vi "PE_IoTSerialProcessor.vi"() -> ()   [LabVIEW 2016]
uses:
  SerialSupport/Serial - Settings.ctl
  SerialSupport/Serial - XON-XOFF Characters.ctl
  SerialSupport/Serial - ASCII Characters.ctl
  <vilib>/Instr/_visa.llb/VISA Configure Serial Port (Instr).vi
  database/database.lvlib
panel:
  in  "持久化开关":bool=TRUE
  in  "参考电阻_AgNW":dbl
  in  "总压降":dbl=65535.0
  in  "参考电阻_ITO":dbl
  in  "JSON parser":T1
  in  "TestId":string
  out "波形图表 2":dynamicdata(graph)
  out "json error":errorcluster caption="JSON Error"
  in  "dataLabel":string
  in  "msg_id":dbl
  out "CtrlCmdMsg":string
  out "串口信息发送持久化":bool=TRUE
  out "串口信息发送":bool=TRUE
  out "UDP发送持久化":bool=TRUE
  out "TCP发送持久化":bool=TRUE
  out "串口接收持久化":bool=TRUE
  in  "串口发送按钮":bool
  in  "终止符":u8=10 format="%.0x"
  in  "终止符时结束写入？":bool=TRUE
  in  "VISA资源名称":refnum<visa-resource-name>="COM3"
  in  "XON/XOFF字符":T2={"XON"=enum."DC1", "XOFF"=enum."DC3"}
  in  "串口设置":T4={"波特率"=115200, "数据位"=8, "校验"=enum."None", "停止位"=10, "流控制"=0} {"流控制" items=["无"=0, "XON/XOFF"=1, "RTS/CTS"=2, "DTR/DSR"=4]; "停止位" items=["1.0"=10, "1.5"=15, "2.0"=20]; "数据位" min=5 max=8 step=1; "波特率" items=["75"=75, "110"=110, "134"=134, "150"=150, "300"=300, "600"=600, "1200"=1200, "1800"=1800, "2400"=2400, "4800"=4800, "7200"=7200, "9600"=9600, "14400"=14400, "19200"=19200, "28800"=28800, "38400"=38400, "56000"=56000, "57600"=57600, "115200"=115200, "128000"=128000, "230400"=230400]}
  in  "终止符时结束读取？":bool=TRUE
  in  "读取":bool=TRUE
  in  "串口停止":bool
  in  "串口发送命令":string="{\"cmd\":\"CT_ON\",\"id\":\"C_FR\",on:true}"
  out "串口信息":string
  in  "串口最大字节":u32=1000
  out "当前指令":string
  # "Smart thermalchromic window monitoring"
  # "Test Information Setting"
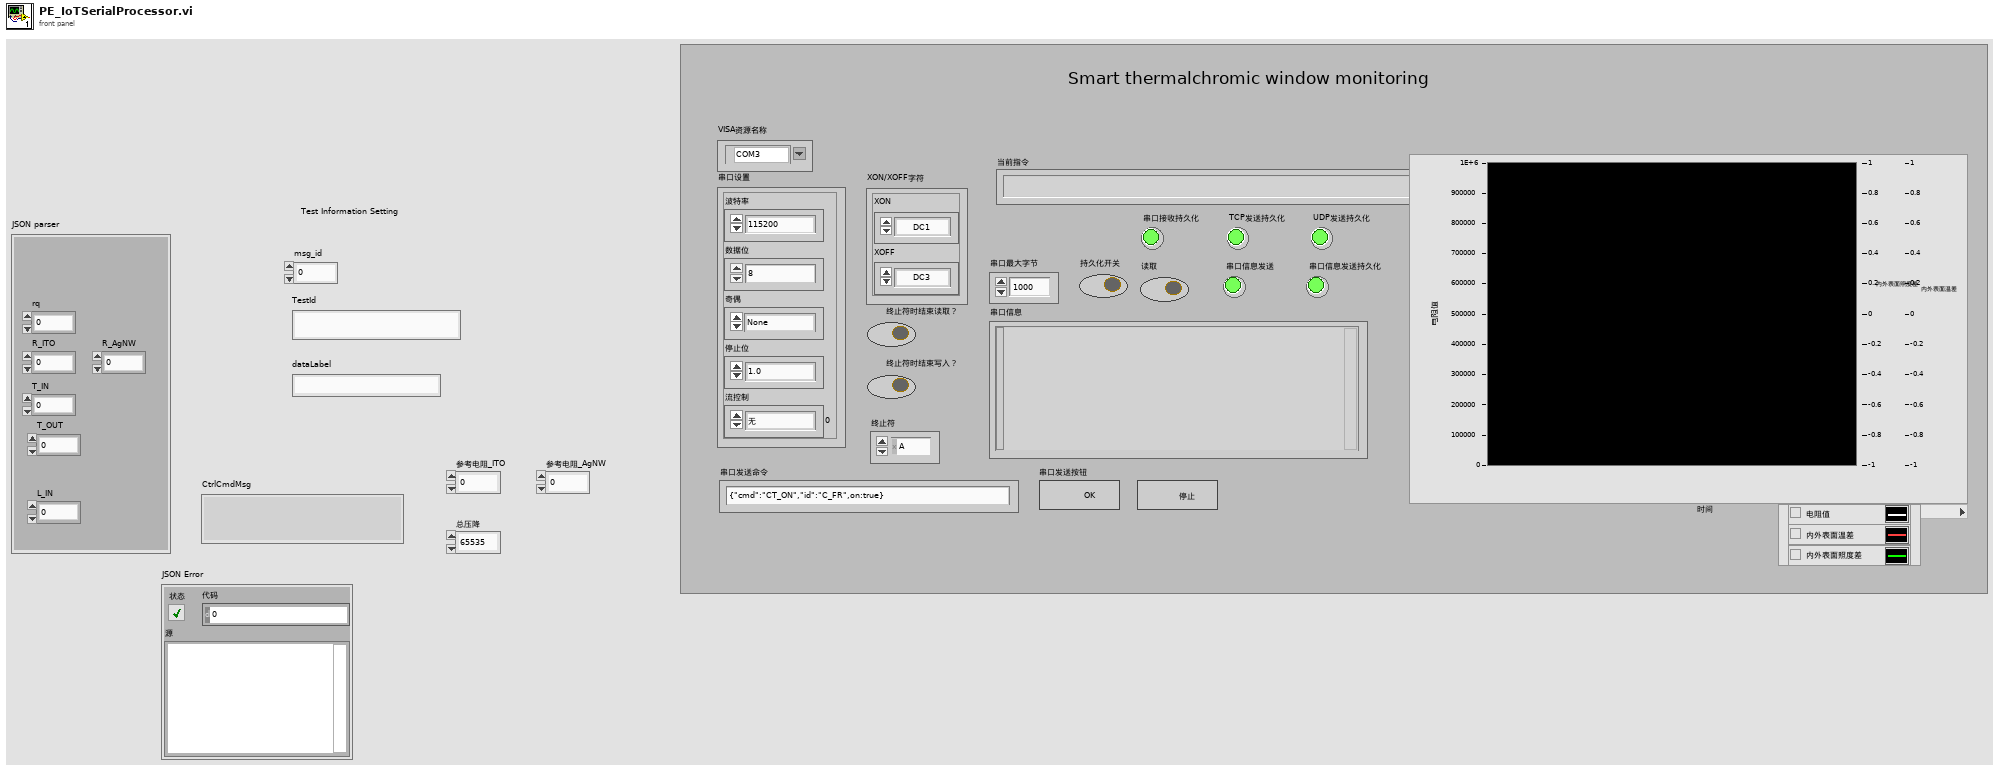
[diagram p1: front panel]
types:
  T1 = cluster{"rq":dbl, "R_ITO":dbl, "T_IN":dbl, "T_OUT":dbl, "R_AgNW":dbl, "L_IN":dbl}
  T2 = typedef "Serial - XON-XOFF Characters.ctl" = cluster{"XON":T3, "XOFF":T3}
  T3 = typedef "Serial - ASCII Characters.ctl" = enum16{"NUL", "SOH", "STX", "ETX", "EOT", "ENQ", "ACK", "BEL", "BS", "HT", "LF", "VT", "FF", "CR", "SO", "SI", "DLE", "DC1", "DC2", "DC3", "DC4", "NAK", "SYN", "ETB", "CAN", "EM", "SUB", "ESC", "FS", "GS", "RS", "US", "SP", "!", "\"", "#", "$", "%", "&", "'", "(", ")", "*", "+", ",", "- (-)", ".", "/", "0", "1", "2", "3", "4", "5", "6", "7", "8", "9", ":", ";", "<", "=", ">", "?", "@", "A", "B", "C", "D", "E", "F", "G", "H", "I", "J", "K", "L", "M", "N", "O", "P", "Q", "R", "S", "T", "U", "V", "W", "X", "Y", "Z", "[", "\\", "]", "^", "_", "`", "a", "b", "c", "d", "e", "f", "g", "h", "i", "j", "k", "l", "m", "n", "o", "p", "q", "r", "s", "t", "u", "v", "w", "x", "y", "z", "{", "|", "}", "~"}
  T4 = typedef "Serial - Settings.ctl" = cluster{"波特率":u32, "数据位":u16, "校验":enum16{"None", "Odd", "Even", "Mark", "Space"}, "停止位":u16, "流控制":u16}
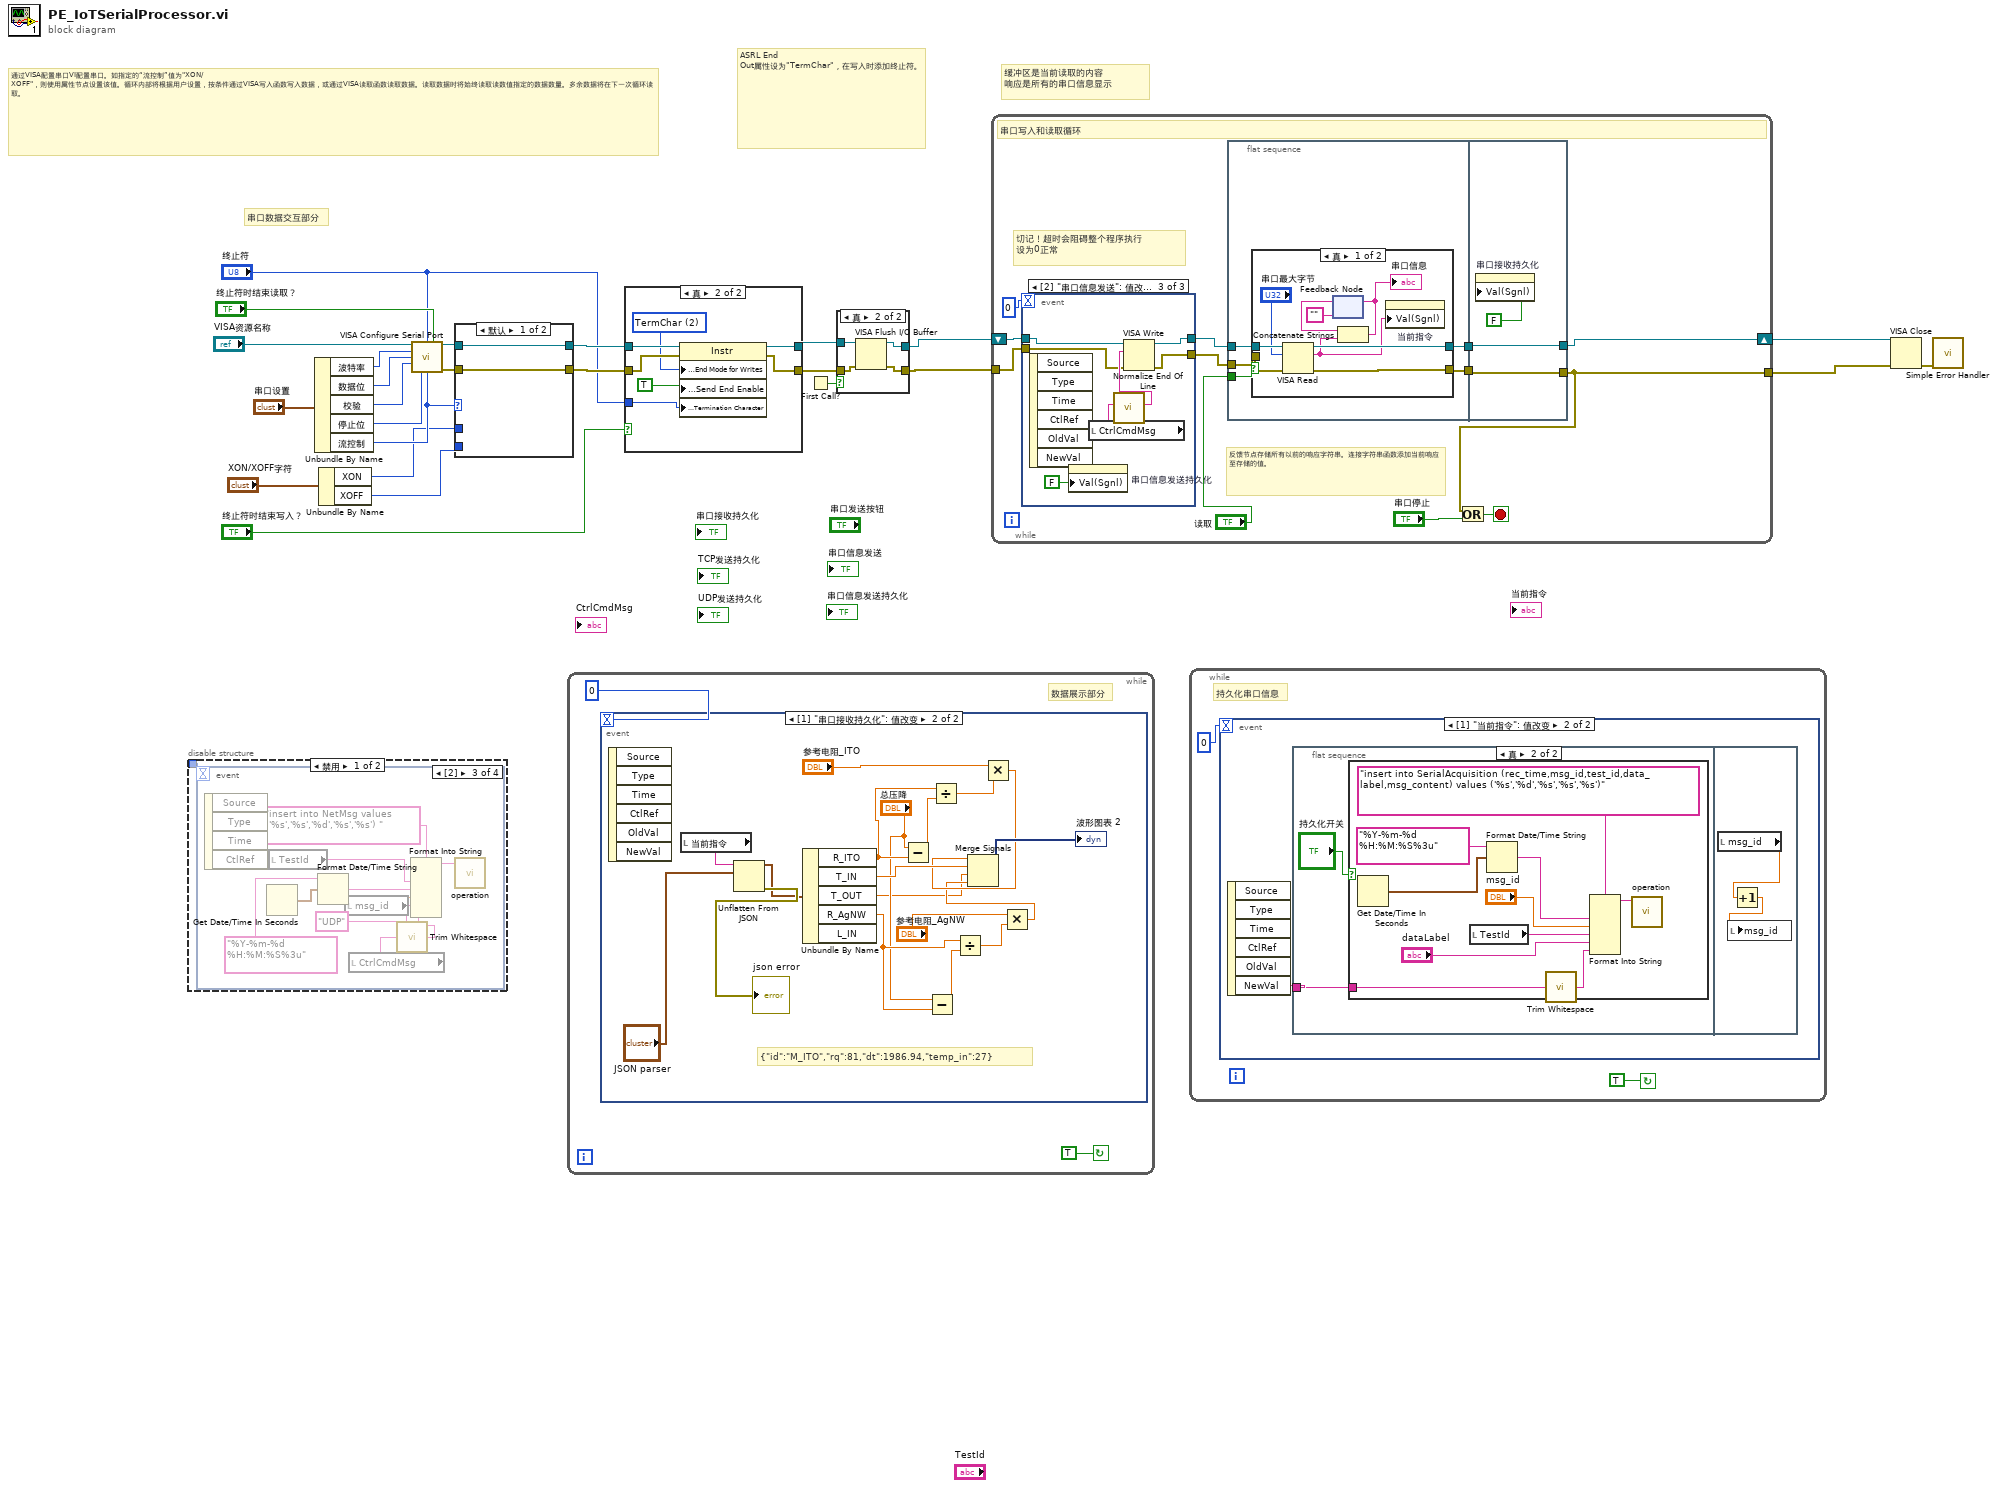
[diagram p0: block diagram]
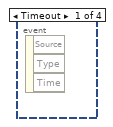
[diagram p2: hidden frame]
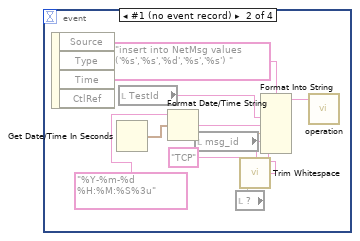
[diagram p3: hidden frame]
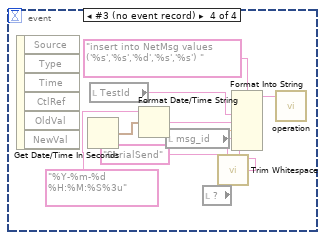
[diagram p4: hidden frame]
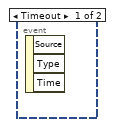
[diagram p6: hidden frame]
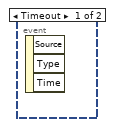
[diagram p8: hidden frame]
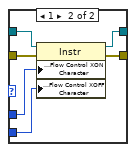
[diagram p11: hidden frame]
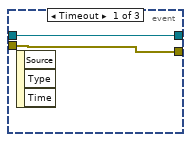
[diagram p13: hidden frame]
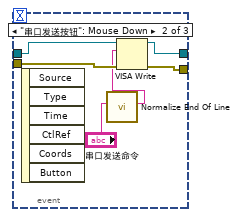
[diagram p14: hidden frame]
diagram:
  # "串口数据交互部分"
  # "缓冲区是当前读取的内容\n响应是所有的串口信息显示"
  # "ASRL End Out属性设为\"TermChar\"，在写入时添加终止符。"
  # "通过VISA配置串口VI配置串口。如指定的“流控制”值为\"XON/XOFF\"，则使用属性节点设置该值。循环内部将根据用户设置，按条件通过VISA写入函数写入数据，或通过VISA读取函数读取数据。读取数据时将始终读取读数值指定的数据数量。多余数据将在下一次循环读取。"
  n1 = disable-structure shown="禁用" {
    disable-tunnel: _ -> [w26 _]
    frame Disabled {
      n2 = event shown="[2]" {
        selector: _ -> [_ _ _ _]
        dyn-events: _ -> [_ _ _ _]
        timeout: w26 -> [_ _ _ _]
        event Timeout {
          n3 = event-data() -> ()  [unwired: 1 in, 3 out]
        }
        event #1 (no event record) {
          n4 = event-data() -> ()  [unwired: 1 in, 4 out]
          n5 = Get Date/Time In Seconds() -> (seconds since 1Jan1904=w33:timestamp)
          n6 = local read "TestId"() -> (w34:string)
          n7 = Format Date/Time String ("格式化日期/时间字符串")(time format string (%c)="%Y-%m-%d %H:%M:%S%3u" ("时间格式字符串(%c)"), seconds (now)=w33) -> (date/time string=w32:string)  [unwired: 1 in]
          n8 = local read "msg_id"() -> (w31:dbl)
          n9 = local read item#-1() -> (w28)
          n10 = call <vilib>:"Trim Whitespace.vi"("string"=w28) -> ("trimmed string"=w27:string)  [unwired: 1 in]
          n11 = Format Into String(format string="insert into NetMsg values ('%s','%s','%d','%s','%s') " ("格式字符串"), w34, w32, w31, "TCP" ("input 4"), w27) -> (resulting string=w35:string)  [unwired: 2 in, 1 out]
          n12 = call "operation.vi"("Command Text"=w35) -> ()  [unwired: 9 in, 1 out]
        }
        event #2 (no event record) {
          n13 = event-data() -> ()  [unwired: 1 in, 4 out]
          n14 = Get Date/Time In Seconds() -> (seconds since 1Jan1904=w43:timestamp)
          n15 = local read "TestId"() -> (w41:string)
          n16 = Format Date/Time String ("格式化日期/时间字符串")(time format string (%c)="%Y-%m-%d %H:%M:%S%3u" ("时间格式字符串(%c)"), seconds (now)=w43) -> (date/time string=w44:string)  [unwired: 1 in]
          n17 = local read "msg_id"() -> (w45:dbl)
          n18 = local read "CtrlCmdMsg"() -> (w38:string)
          n19 = call <vilib>:"Trim Whitespace.vi"("string"=w38) -> ("trimmed string"=w37:string)  [unwired: 1 in]
          n20 = Format Into String(format string="insert into NetMsg values ('%s','%s','%d','%s','%s') " ("格式字符串"), w41, w44, w45, "UDP" ("input 4"), w37) -> (resulting string=w40:string)  [unwired: 2 in, 1 out]
          n21 = call "operation.vi"("Command Text"=w40) -> ()  [unwired: 9 in, 1 out]
        }
        event #3 (no event record) {
          n22 = event-data() -> ()  [unwired: 1 in, 6 out]
          n23 = Get Date/Time In Seconds() -> (seconds since 1Jan1904=w53:timestamp)
          n24 = local read "TestId"() -> (w52:string)
          n25 = Format Date/Time String ("格式化日期/时间字符串")(time format string (%c)="%Y-%m-%d %H:%M:%S%3u" ("时间格式字符串(%c)"), seconds (now)=w53) -> (date/time string=w54:string)  [unwired: 1 in]
          n26 = local read "msg_id"() -> (w55:dbl)
          n27 = local read item#-1() -> (w49)
          n28 = call <vilib>:"Trim Whitespace.vi"("string"=w49) -> ("trimmed string"=w48:string)  [unwired: 1 in]
          n29 = Format Into String(format string="insert into NetMsg values ('%s','%s','%d','%s','%s') " ("格式字符串"), w52, w54, w55, "SerialSend" ("input 4"), w48) -> (resulting string=w51:string)  [unwired: 2 in, 1 out]
          n30 = call "operation.vi"("Command Text"=w51) -> ()  [unwired: 9 in, 1 out]
        }
      }
    }
    frame Enabled {
    }
  }
  n31 = Unbundle By Name("串口设置") -> ("波特率"=w18:u32, "数据位"=w19:u16, "校验"=w20:enum16{"None", "Odd", "Even", "Mark", "Space"}, "停止位"=w21:u16, "流控制"=w13:u16)
  n32 = Unbundle By Name("XON/XOFF字符") -> ("XON"=w12:T3, "XOFF"=w11:T3)
  n33 = call-poly "VISA Configure Serial Port"("VISA resource name"="VISA资源名称", "termination char\n(0xA = '\\n' = LF)"="终止符", "Enable Termination\nChar (T)"="终止符时结束读取？", "baud rate (9600)"=w18, "data bits (8)"=w19, "parity (0:none)"=w20, "stop bits (10: 1 bit)"=w21, "flow control (0:none)"=w13) -> ("VISA resource name out"=w22:refnum<visa-resource-name>, "error out"=w23:errorcluster)  [unwired: 2 in, 4 out]
  n34 = case shown="默认" w13 {
    tunnel: [w57 w64] -> w10
    tunnel: [w58 w63] -> w9
    tunnel: w23 -> [w57 w62]
    tunnel: w22 -> [w58 w61]
    tunnel: w12 -> [_ w60]
    tunnel: w11 -> [_ w59]
    frame Default {
    }
    frame 1 {
      n35 = property class="Instr"(reference=w61, error in=w62, "Serial Settings:Flow Control XON Character"=w60, "Serial Settings:Flow Control XOFF Character"=w59) -> (reference out=w63:refnum<visa-resource-name>, error out=w64:errorcluster)
    }
  }
  n36 = while {
    stop <- TRUE continue-if-true
    # "数据展示部分"
    n37 = event shown="[1] \"串口接收持久化\": 值改变" {
      selector: _ -> [_ _]
      dyn-events: _ -> [_ _]
      timeout: 0 -> [_ _]
      event Timeout {
        n38 = event-data() -> ()  [unwired: 1 in, 3 out]
      }
      event "串口接收持久化": Value Change {
        # "{\"id\":\"M_ITO\",\"rq\":81,\"dt\":1986.94,\"temp_in\":27}"
        n39 = event-data() -> ()  [unwired: 1 in, 6 out]
        n40 = local read "当前指令"() -> (w84:string)
        n41 = Unflatten From JSON(JSON string=w84, type and defaults="JSON parser") -> (value=w81:T1, error out=→"json error":errorcluster)  [unwired: 5 in]
        n42 = Unbundle By Name(w81) -> ("R_ITO"=w78:dbl, "T_IN"=w80:dbl, "T_OUT"=w67:dbl, "R_AgNW"=w70:dbl)  [unwired: 1 out]
        n43 = Subtract(x="总压降", y=w78) -> (x-y=w77:dbl)
        n44 = Subtract(x="总压降", y=w70) -> (x-y=w73:dbl)
        n45 = Divide(x=w78, y=w77) -> (x/y=w76:dbl)
        n46 = Divide(x=w70, y=w73) -> (x/y=w72:dbl)
        n47 = Multiply(x="参考电阻_ITO", y=w76) -> (x*y=w74:dbl)
        n48 = Multiply(x="参考电阻_AgNW", y=w72) -> (x*y=w68:dbl)
        n49 = Merge Signals(w74, w80, w67, w68) -> (→"波形图表 2":dynamicdata)
      }
    }
  }
  n50 = case shown="真" "终止符时结束写入？" {
    tunnel: w9 -> [w85 w93]
    tunnel: w10 -> [w86 w92]
    tunnel: [w85 w91] -> w6
    tunnel: [w86 w90] -> w5
    tunnel: "终止符" -> [_ w88]
    frame False {
    }
    frame True {
      w89 = u16 2 items=["None", "LastBit", "TermChar", "Break"] ("Serial Settings:Serial End Mode for Writes")
      n51 = property class="Instr"(reference=w93, error in=w92, "Serial Settings:End Mode for Writes"=w89, "Message Based Settings:Send End Enable"=TRUE, "Message Based Settings:Termination Character"=w88) -> (reference out=w91:refnum<visa-resource-name>, error out=w90:errorcluster)
    }
  }
  n52 = First Call?() -> (First Call?: T/F=w2:bool)
  n53 = case shown="真" w2 {
    tunnel: w6 -> [w95 w99]
    tunnel: w5 -> [w94 w98]
    tunnel: [w95 w97] -> w4
    tunnel: [w94 w96] -> w3
    frame False {
    }
    frame True {
      n54 = VISA Flush I/O Buffer(VISA resource name=w99, error in (no error)=w98) -> (VISA resource name out=w97:refnum<visa-resource-name>, error out=w96:errorcluster)  [unwired: 1 in]
    }
  }
  n55 = while {
    shift-right: [w101] -> w14
    shift-left: w4 -> [w106]
    tunnel: w3 -> [w108]
    tunnel: [w100] -> w1
    stop <- w110 stop-if-true
    # "反馈节点存储所有以前的响应字符串。连接字符串函数添加当前响应至存储的值。"
    # "切记！超时会阻碍整个程序执行\n设为0正常"
    # "串口写入和读取循环"
    n56 = event shown="[2] \"串口信息发送\": 值改变" {
      selector: _ -> [_ _ _]
      dyn-events: _ -> [_ _ _]
      timeout: 0 -> [_ _ _]
      tunnel: w108 -> [w131 w138 w141]
      tunnel: [w131 w137 w142] -> w107
      tunnel: w106 -> [w132 w136 w144]
      tunnel: [w132 w135 w143] -> w105
      event Timeout {
        n57 = event-data() -> ()  [unwired: 1 in, 3 out]
      }
      event "串口发送按钮": Mouse Down {
        n58 = event-data() -> ()  [unwired: 1 in, 6 out]
        n59 = call <vilib>:"Normalize End Of Line.vi"("string in"="串口发送命令") -> ("string out"=w133:string)  [unwired: 7 in]
        n60 = VISA Write(VISA resource name=w136, write buffer=w133, error in (no error)=w138) -> (VISA resource name out=w135:refnum<visa-resource-name>, error out=w137:errorcluster)  [unwired: 1 out]
      }
      event "串口信息发送": Value Change {
        n61 = event-data() -> ()  [unwired: 1 in, 6 out]
        n62 = property on="串口信息发送持久化" class="Bool (严格)"("Val(Sgnl)"=FALSE ("Value (Signaling)")) -> ()  [unwired: 2 in, 2 out]
        n63 = local read "CtrlCmdMsg"() -> (w140:string)
        n64 = call <vilib>:"Normalize End Of Line.vi"("string in"=w140) -> ("string out"=w145:string)  [unwired: 7 in]
        n65 = VISA Write(VISA resource name=w144, write buffer=w145, error in (no error)=w141) -> (VISA resource name out=w143:refnum<visa-resource-name>, error out=w142:errorcluster)  [unwired: 1 out]
      }
    }
    n66 = flat-sequence {
      tunnel: "读取" -> [w115]
      tunnel: w107 -> [w113]
      tunnel: w105 -> [w112]
      tunnel: [w116] -> w103
      tunnel: [w114] -> w102
      tunnel: w103 -> [w129]
      tunnel: w102 -> [w128]
      tunnel: [w129] -> w101
      tunnel: [w128] -> w100
      frame #0 {
        n67 = case shown="真" w115 {
          tunnel: [w123 w127] -> w116
          tunnel: w112 -> [w125 w127]
          tunnel: [w121 w126] -> w114
          tunnel: w113 -> [w124 w126]
          frame True {
            n68 = VISA Read(VISA resource name=w125, byte count="串口最大字节", error in (no error)=w124) -> (VISA resource name out=w123:refnum<visa-resource-name>, read buffer=w117:string, error out=w121:errorcluster)  [unwired: 1 out]
            n69 = feedback #1("") -> (w120:string)
            n70 = Concatenate Strings(w120, w117) -> (w119:string)
            "串口信息" <- w119
            n71 = feedback-in #1(w119) -> ()
            n72 = property on="当前指令" class="Str"("Val(Sgnl)"=w117) -> ()  [unwired: 2 in, 2 out]
          }
          frame False {
          }
        }
      }
      frame #1 {
        n73 = property on="串口接收持久化" class="Bool (严格)"("Val(Sgnl)"=FALSE ("Value (Signaling)")) -> ()  [unwired: 2 in, 2 out]
      }
    }
    n74 = Or(x=w100, y="串口停止") -> (x .or. y?=w110:bool)
  }
  n75 = while {
    stop <- TRUE continue-if-true
    # "持久化串口信息"
    n76 = event shown="[1] \"当前指令\": 值改变" {
      selector: _ -> [_ _]
      dyn-events: _ -> [_ _]
      timeout: 0 -> [_ _]
      event Timeout {
        n77 = event-data() -> ()  [unwired: 1 in, 3 out]
      }
      event "当前指令": Value Change {
        n78 = event-data() -> ("NewVal"=w148:string)  [unwired: 1 in, 5 out]
        n79 = flat-sequence {
          tunnel: w148 -> [w150]
          frame #0 {
            n80 = case shown="真" "持久化开关" {
              tunnel: w150 -> [_ w152]
              frame False {
              }
              frame True {
                n81 = Get Date/Time In Seconds() -> (seconds since 1Jan1904=w158:timestamp)
                n82 = local read "TestId"() -> (w154:string)
                n83 = Format Date/Time String ("格式化日期/时间字符串")(time format string (%c)="%Y-%m-%d %H:%M:%S%3u" ("时间格式字符串(%c)"), seconds (now)=w158) -> (date/time string=w155:string)  [unwired: 1 in]
                n84 = call <vilib>:"Trim Whitespace.vi"("string"=w152) -> ("trimmed string"=w156:string)  [unwired: 1 in]
                n85 = Format Into String(format string="insert into SerialAcquisition (rec_time,msg_id,test_id,data_label,msg_content) values ('%s','%d','%s','%s','%s')" ("格式字符串"), w155, "msg_id", w154, "dataLabel", w156) -> (resulting string=w157:string)  [unwired: 2 in, 1 out]
                n86 = call "operation.vi"("Command Text"=w157) -> ()  [unwired: 9 in, 1 out]
              }
            }
          }
          frame #1 {
            n87 = local read "msg_id"() -> (w162:dbl)
            n88 = Increment(x=w162) -> (x+1=w161:dbl)
            n89 = local write "msg_id"(w161) -> ()
          }
        }
      }
    }
  }
  n90 = VISA Close(VISA resource name=w14, error in (no error)=w1) -> (error out=w15:errorcluster)
  n91 = call <vilib>:"Simple Error Handler.vi"("error in (no error)"=w15) -> ()  [unwired: 1 in, 8 out]
